vi "CAENHV Get Sys Prop String.vi"(8 "error in (no error)":errorcluster, 10 "PropName":string, 11 "handle":i32) -> (0 "error out":errorcluster, 3 "Result":string)   [LabVIEW 2009, in "CAENHVWrapper.lvlib"]
doc: "CAENHVLIB_API CAENHVRESULT CAENHV_GetSysProp(int handle, \n const char *PropName, void *Result);"
uses:
  <userlib>/CAENHVWrapper/CAENHVWrapper.lvlib
  <vilib>/Utility/error.llb/whitespace.ctl
  <userlib>/CAENHVWrapper/CAENHVWrapper.dll
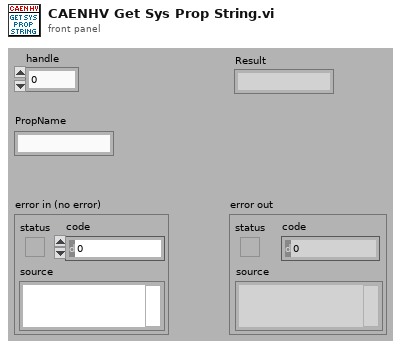
[diagram p1: front panel]
types:
  T1 = typedef "CAENHVWrapper.lvlib/SYSPROP_TYPE.ctl" = enum32{"SYSPROP_TYPE_STR", "SYSPROP_TYPE_REAL", "SYSPROP_TYPE_UINT2", "SYSPROP_TYPE_UINT4", "SYSPROP_TYPE_INT2", "SYSPROP_TYPE_INT4", "SYSPROP_TYPE_BOOLEAN"}
  T2 = typedef "whitespace.ctl" = u16
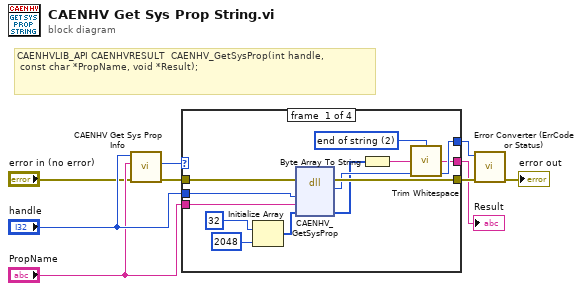
[diagram p0: block diagram]
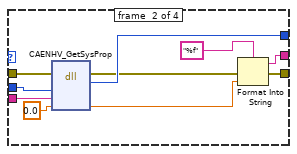
[diagram p2: hidden frame]
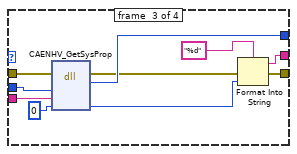
[diagram p3: hidden frame]
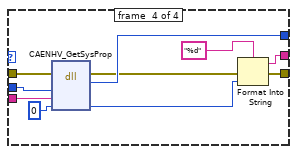
[diagram p4: hidden frame]
diagram:
  # "CAENHVLIB_API CAENHVRESULT  CAENHV_GetSysProp(int handle, \n const char *PropName, void *Result);"
  n1 = call <userlib>:"CAENHV Get Sys Prop Info.vi"("error in (no error)"="error in (no error)", "PropName"="PropName", "handle"="handle") -> ("error out"=w2:errorcluster, "PropType"=w3:T1)  [unwired: 6 in, 1 out]
  n2 = case shown="\"SYSPROP_TYPE_STR\", Default" w3 {
    tunnel: [w17 w31 w41 w51] -> w9
    tunnel: [w18 w22 w32 w42] -> w8
    tunnel: "handle" -> [w20 w30 w40 w50]
    tunnel: "PropName" -> [w19 w29 w39 w49]
    tunnel: w2 -> [w21 w28 w38 w48]
    tunnel: [w11 w24 w34 w44] -> w1
    frame #0 {
      w10 = T2 2 items=["both", "start of string", "end of string"] ("location (both)")
      n3 = Initialize Array(u8 32 ("element"), 2048 ("dimension size")) -> (w14:u8[])
      n4 = dll-call lib="C:/Program Files/National Instruments/LabVIEW 2009/user.lib/CAENHVWrapper/CAENHVWrapper.*" fn="CAENHV_GetSysProp"(error in=w21, "handle"=w20, "PropName"=w19, "Result"=w14) -> (error out=w18:errorcluster, "return type"=w17:i32, "Result"=w13:u8[])  [unwired: 4 in, 1 out]
      n5 = Byte Array To String(unsigned byte array=w13) -> (string=w12:string)
      n6 = call <vilib>:"Trim Whitespace.vi"("string"=w12, "location (both)"=w10) -> ("trimmed string"=w11:string)
    }
    frame #1 {
      n7 = dll-call lib="C:/Program Files/National Instruments/LabVIEW 2009/user.lib/CAENHVWrapper/CAENHVWrapper.*" fn="CAENHV_GetSysProp"(error in=w28, "handle"=w30, "PropName"=w29, "Result"=sgl 0.0) -> (error out=w23:errorcluster, "return type"=w31:i32, "Result"=w26:sgl)  [unwired: 4 in, 1 out]
      n8 = Format Into String(format string="%f", error in=w23, w26) -> (resulting string=w24:string, error out=w22:errorcluster)  [unwired: 1 in]
    }
    frame #2 {
      n9 = dll-call lib="C:/Program Files/National Instruments/LabVIEW 2009/user.lib/CAENHVWrapper/CAENHVWrapper.*" fn="CAENHV_GetSysProp"(error in=w38, "handle"=w40, "PropName"=w39, "Result"=u16 0) -> (error out=w33:errorcluster, "return type"=w41:i32, "Result"=w36:u16)  [unwired: 4 in, 1 out]
      n10 = Format Into String(format string="%d", error in=w33, w36) -> (resulting string=w34:string, error out=w32:errorcluster)  [unwired: 1 in]
    }
    frame #3 {
      n11 = dll-call lib="C:/Program Files/National Instruments/LabVIEW 2009/user.lib/CAENHVWrapper/CAENHVWrapper.*" fn="CAENHV_GetSysProp"(error in=w48, "handle"=w50, "PropName"=w49, "Result"=i16 0) -> (error out=w43:errorcluster, "return type"=w51:i32, "Result"=w46:i16)  [unwired: 4 in, 1 out]
      n12 = Format Into String(format string="%d", error in=w43, w46) -> (resulting string=w44:string, error out=w42:errorcluster)  [unwired: 1 in]
    }
  }
  "Result" <- w1
  n13 = call <userlib>:"Error Converter (ErrCode or Status).vi"("error in (no error)"=w8, "error code"=w9) -> ("error out"=→"error out":errorcluster)  [unwired: 9 in]
